vi "Process.vi"(8 "error in":errorcluster, 11 "System":refnum<class "System.lvclass">) -> (0 "error out":errorcluster, 3 "System out":refnum<class "System.lvclass">)   [LabVIEW 2014, in "System.lvclass"]
doc: "JKI State Machine Objects (SMO) 1.4.0.57\nJKI - JKI\nCopyright (c) 2018, JKI"
uses:
  System.lvclass
  <vilib>/JKI/JKI SMO/SMO/Typedefs/Parent Call--Enum.ctl
  Pump class/Pump State - cluster.ctl
  System.lvclass/System.ctl
  Pump class/Pump.lvclass/Pump.ctl
  <vilib>/JKI/JKI SMO/SMO/SMO.lvclass
  Pump class/Pump.lvclass
panel:
  in  "Speed Command":dbl
  in  "Change Pump Speed":bool
  out "Pump State":T1(graph)
  # "For instructions on how to use the JKI State Machine Objects, examples and video tutorials, visit:\nhttp://jki.net/state-machine-objects/\n\nJKI State Machine Objects™\nhttp://jki.net/state-machine-objects/\nCopyright (C) 2005-2015, JKI <info@jki.net>\nALL RIGHTS RESERVED"
  # "SYSTEM PROCESS USER INTERFACE"
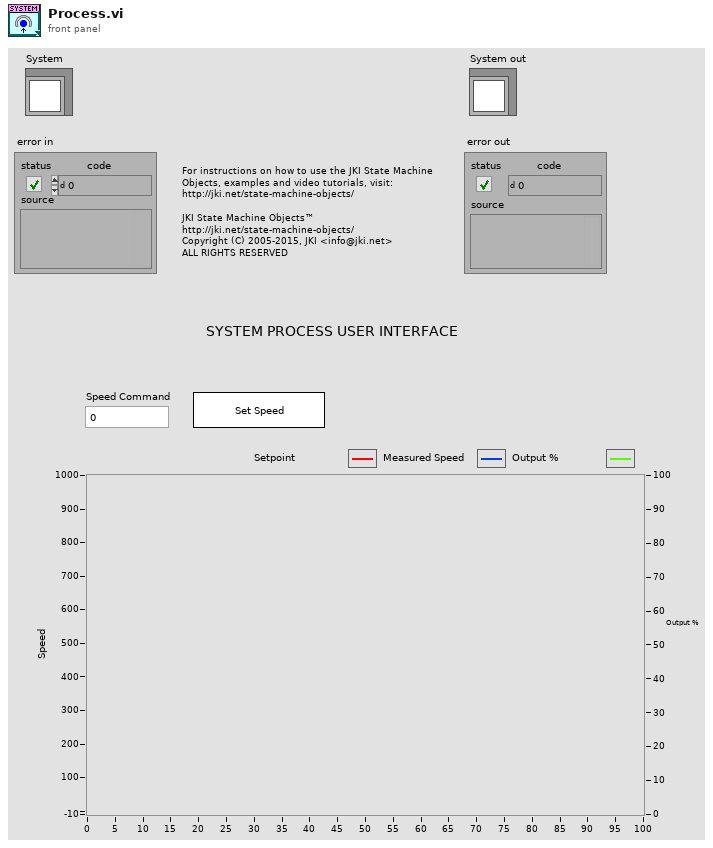
[diagram p1: front panel]
types:
  T1 = typedef "Pump.lvclass/Pump State - cluster.ctl" = cluster{"Pump Setpoint":dbl, "Pump Speed":dbl, "Output %":dbl}
  T2 = typedef "SMO.lvclass/Parent Call--Enum.ctl" = enum16{"Allows parent to run", "Does not request parent to run"}
  T3 = enum32{"invalid app kind", "Development System", "Run Time System", "Student Edition", "Embedded LabVIEW", "Evaluation", "Custom"}
  T4 = enum32{"Invalid", "Standard", "Closed", "Hidden", "Minimized", "Maximized"}
  T5 = cluster{"Core":cluster{"Current VI Reference":refnum<vi>, "Close Panel on Exit?":bool, "error":errorcluster}, "Self Reference":refnum<class "System.lvclass">}
  T6 = cluster{"Current VI Reference":refnum<vi>, "Close Panel on Exit?":bool, "error":errorcluster}
  T7 = typedef "SMO.lvclass/Protected Events.ctl" = cluster{"StopProcesses":refnum<user-event>, "AbortProcesses":refnum<user-event>, "Config Changed":refnum<user-event>, "Dependency":refnum<user-event>}
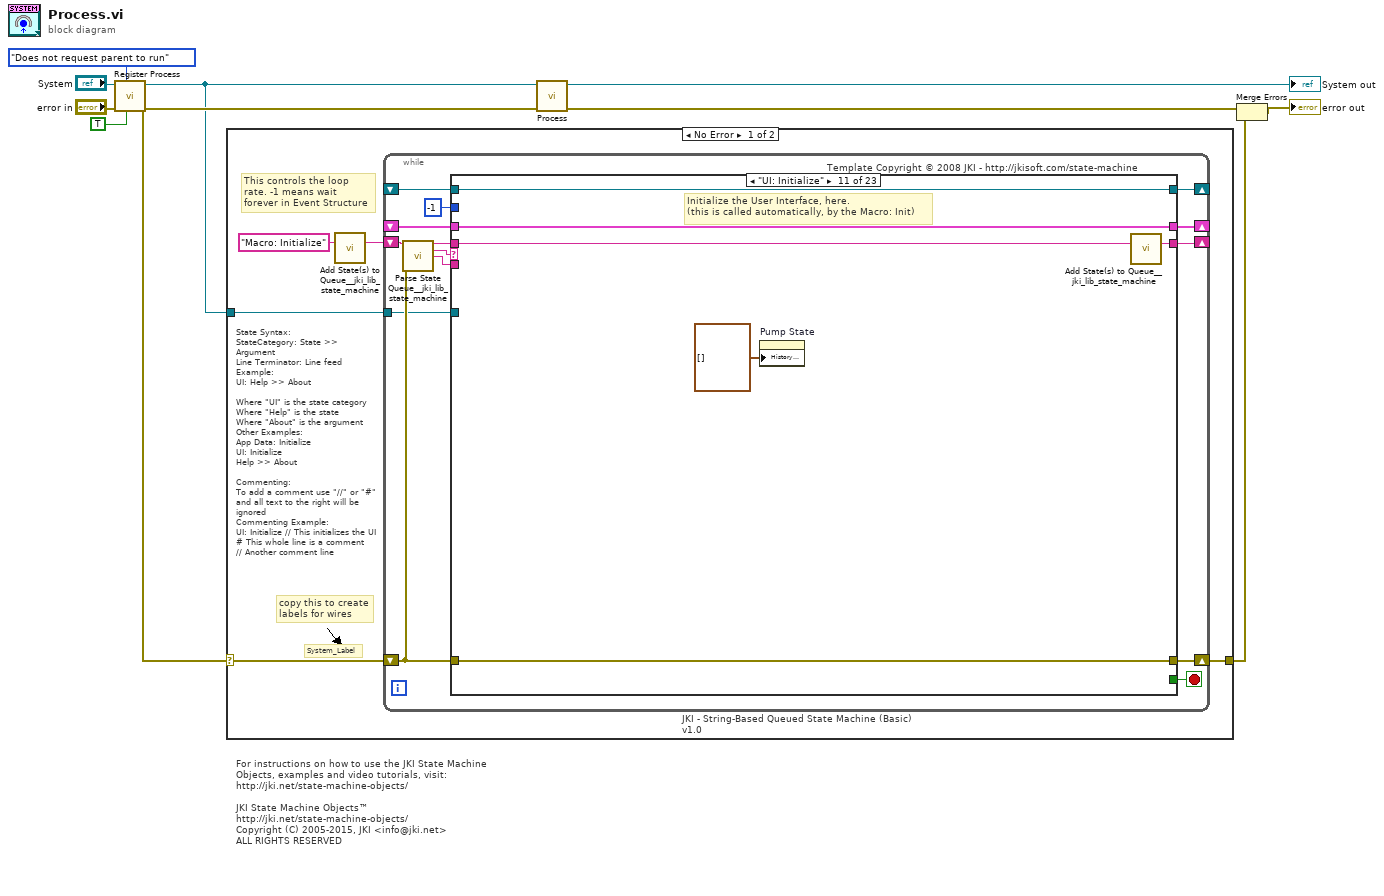
[diagram p0: block diagram]
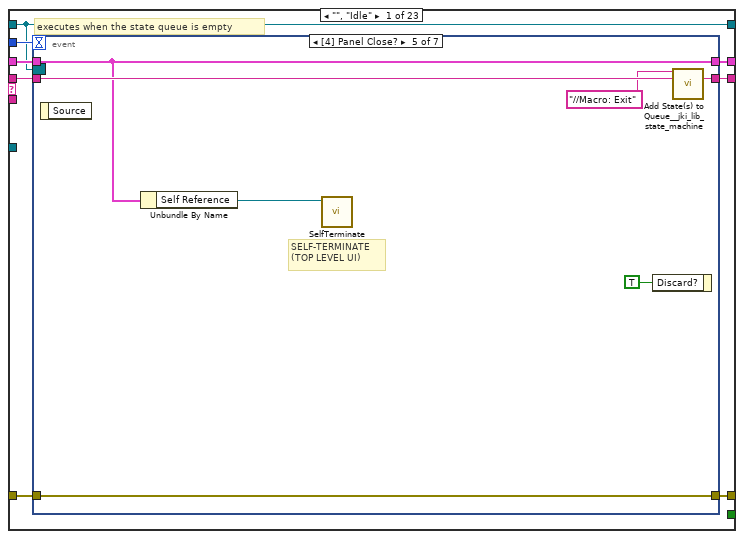
[diagram p2: hidden frame]
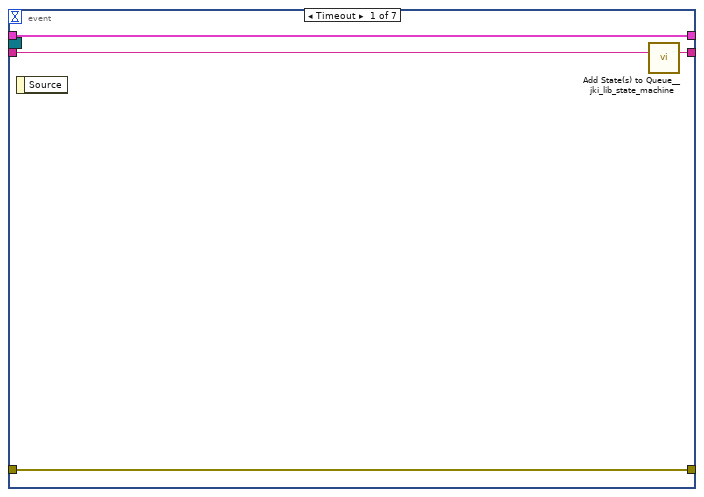
[diagram p3: hidden frame]
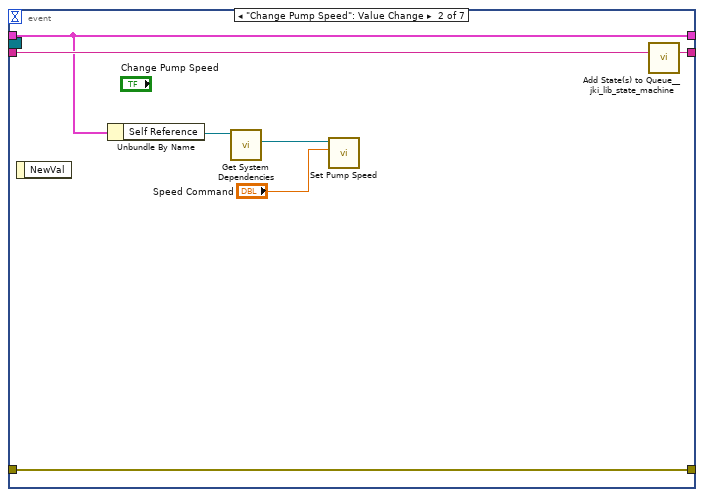
[diagram p4: hidden frame]
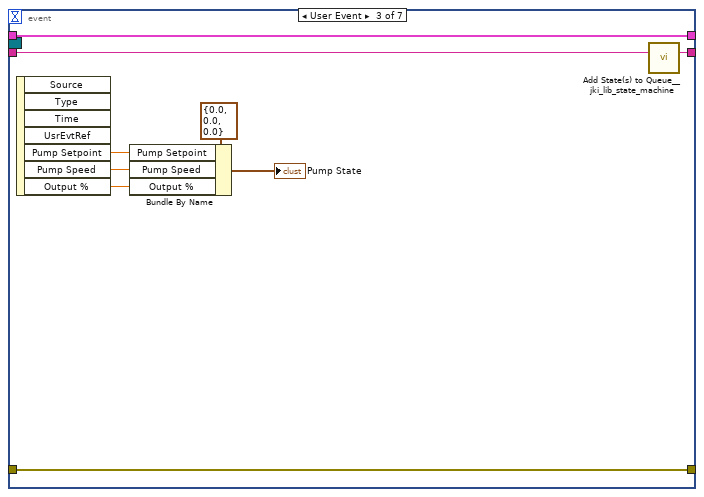
[diagram p5: hidden frame]
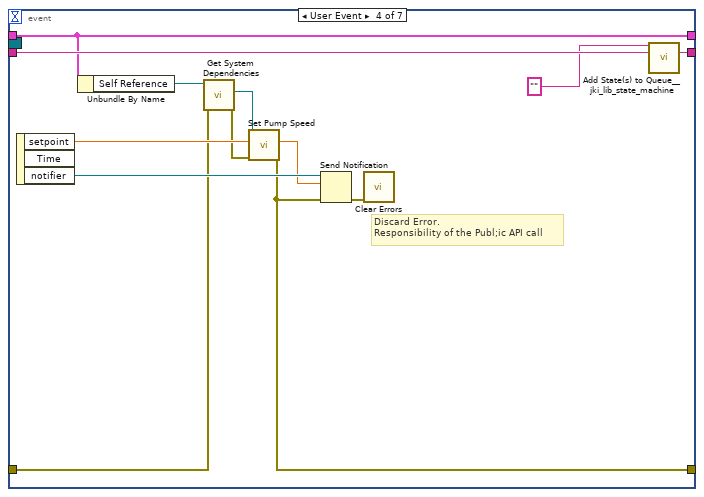
[diagram p6: hidden frame]
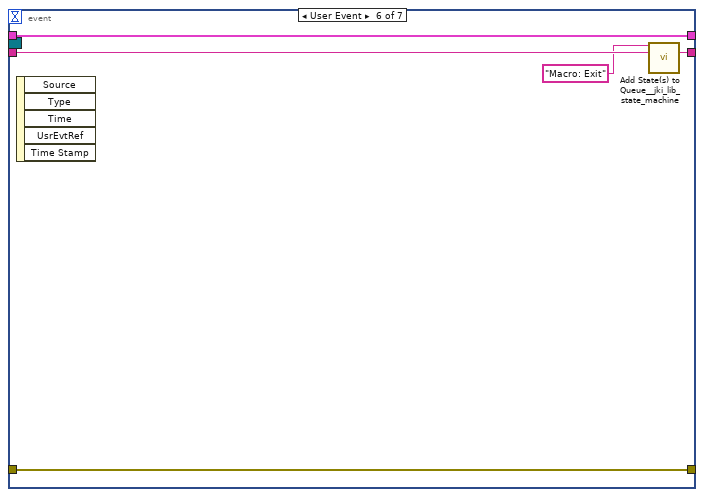
[diagram p7: hidden frame]
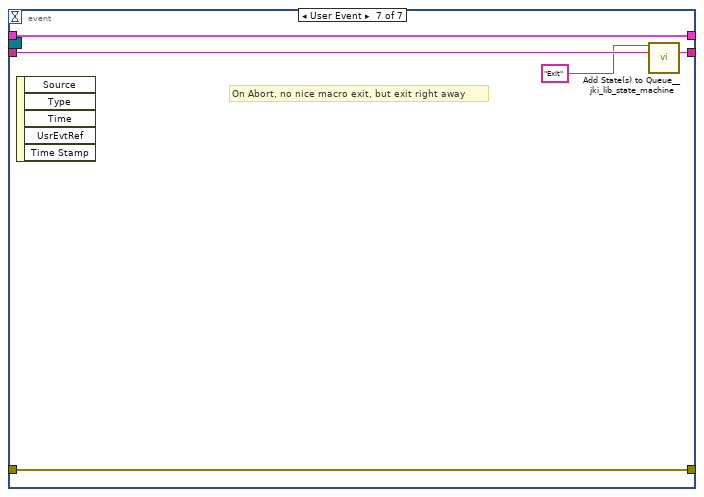
[diagram p8: hidden frame]
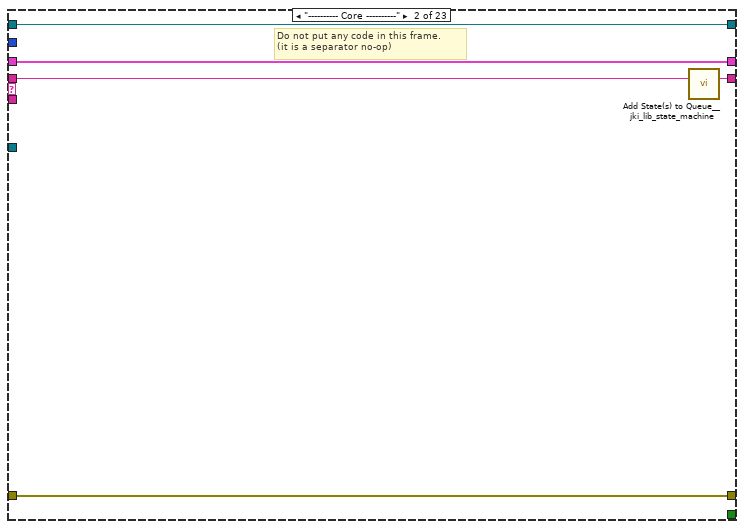
[diagram p9: hidden frame]
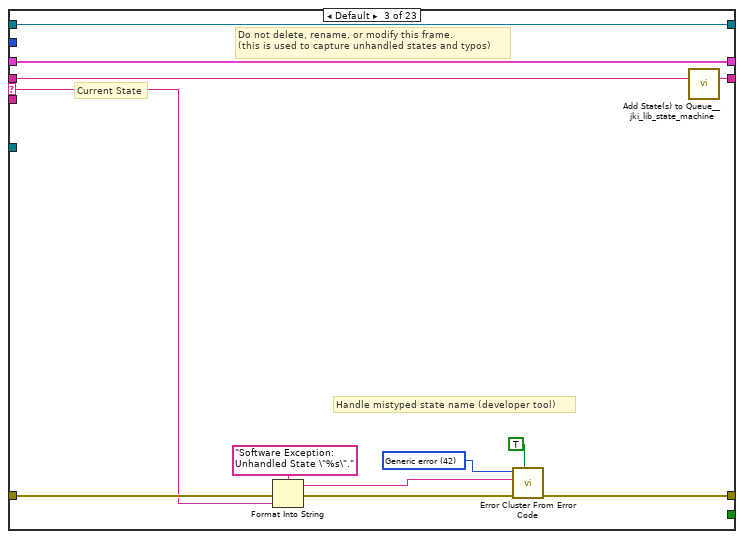
[diagram p10: hidden frame]
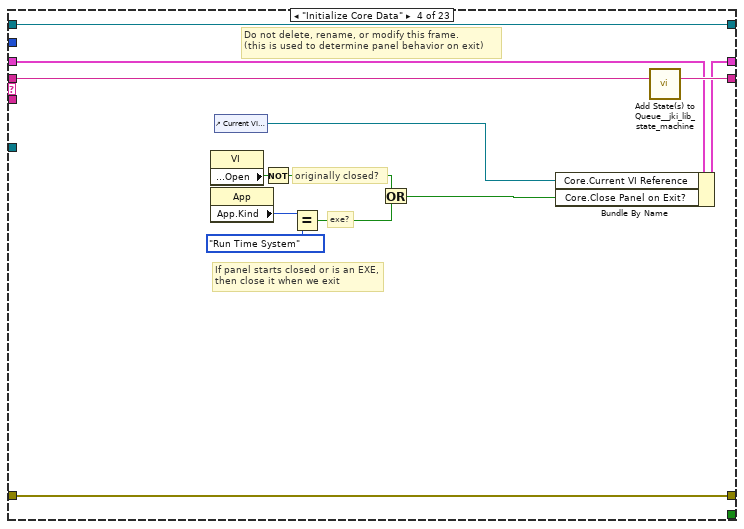
[diagram p11: hidden frame]
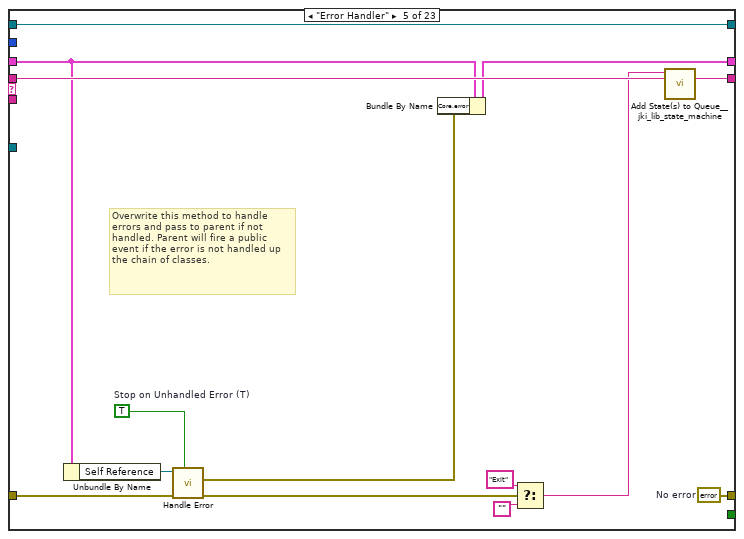
[diagram p12: hidden frame]
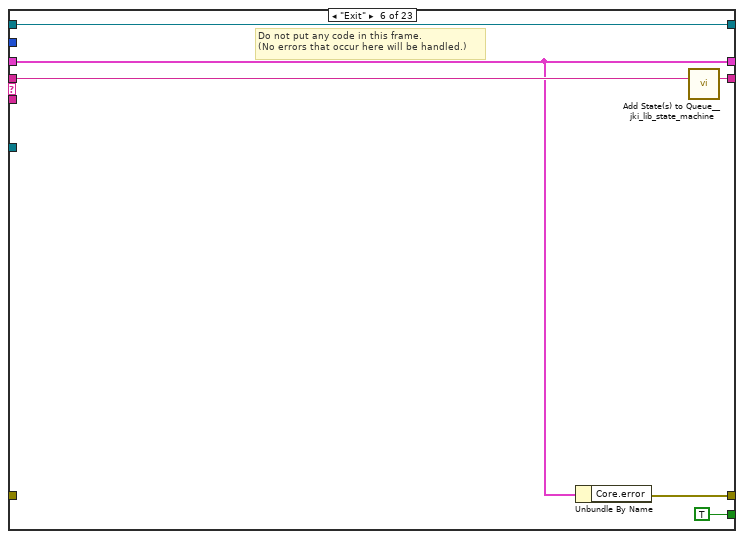
[diagram p13: hidden frame]
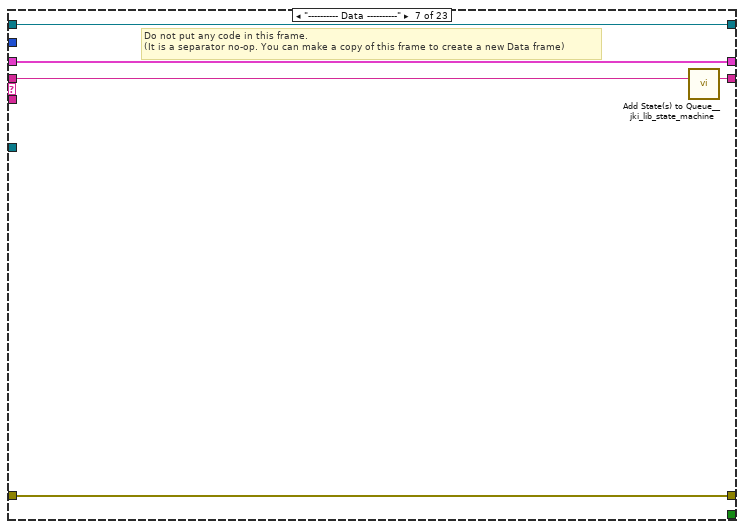
[diagram p14: hidden frame]
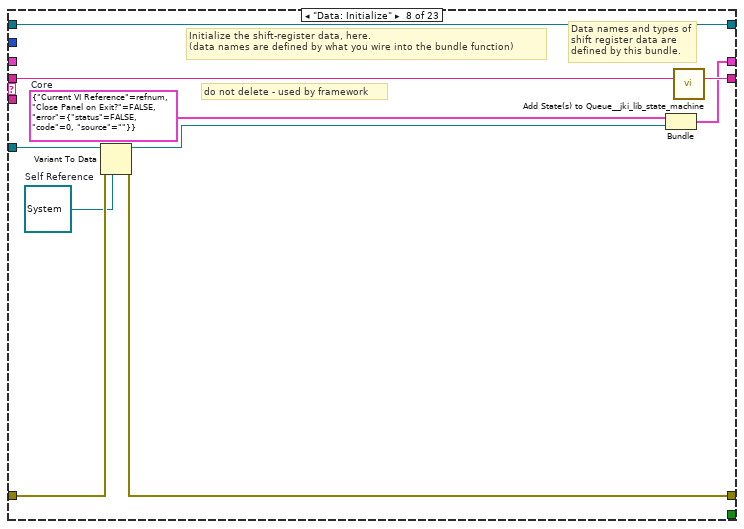
[diagram p15: hidden frame]
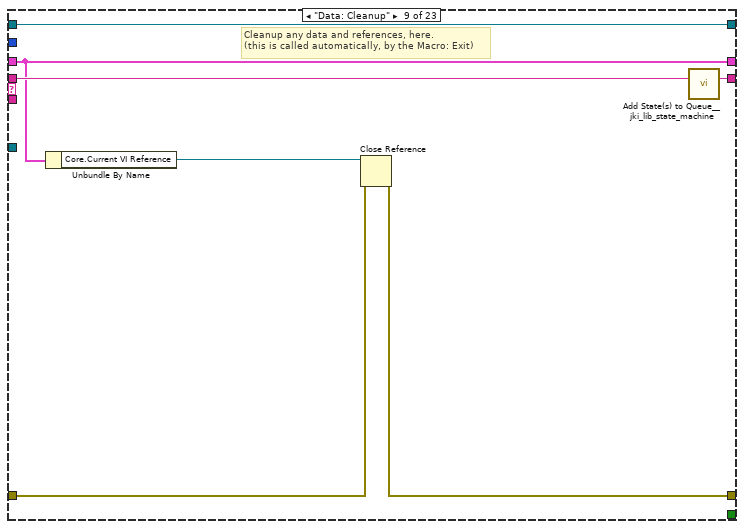
[diagram p16: hidden frame]
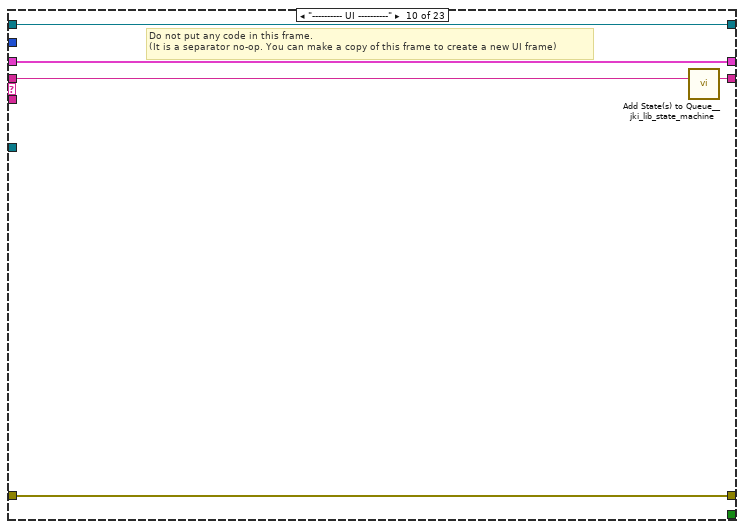
[diagram p17: hidden frame]
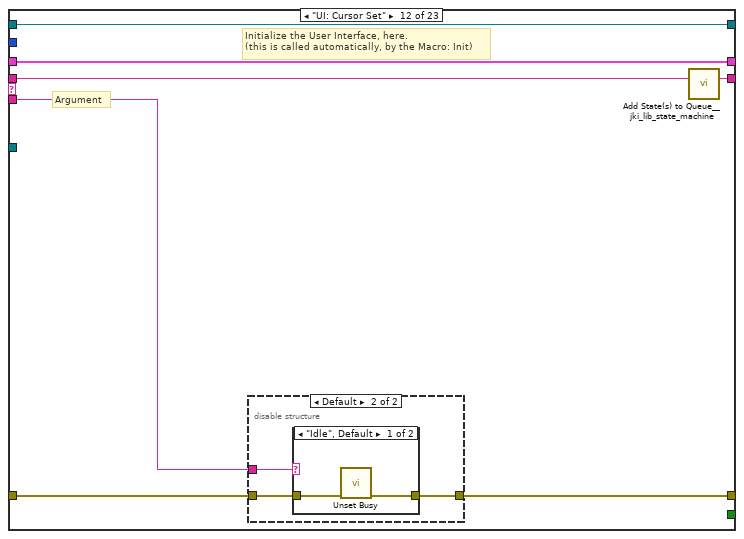
[diagram p18: hidden frame]
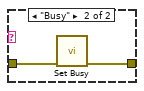
[diagram p20: hidden frame]
diagram:
  # "For instructions on how to use the JKI State Machine Objects, examples and video tutorials, visit:\nhttp://jki.net/state-machine-objects/\n\nJKI State Machine Objects™\nhttp://jki.net/state-machine-objects/\nCopyright (C) 2005-2015, JKI <info@jki.net>\nALL RIGHTS RESERVED"
  n1 = call <vilib>:"Register Process.vi"("Forces Self to Run (F)"=TRUE, "Parent Call"=Parent_Call--Enum."Does not request parent to run", "error in (no error)"="error in", "SMO"="System") -> ("error out"=w10:errorcluster, "SMO out"=w9:refnum<class "System.lvclass">)  [unwired: 6 in]
  n2 = case shown="No Error" w10 {
    selector: w10 -> [w12 w302]
    tunnel: w9 -> [w13 _]
    tunnel: [w11 w302] -> w7
    frame No Error {
      # "State Syntax:\nStateCategory: State >> Argument\nLine Terminator: Line feed\nExample:\nUI: Help >> About\n\nWhere \"UI\" is the state category\nWhere \"Help\" is the state\nWhere \"About\" is the argument\nOther Examples:\nApp Data: Initialize\nUI: Initialize\nHelp >> About\n\nCommenting:\nTo add a comment use \"//\" or \"#\" and all text to the right will be ignored\nCommenting Example:\nUI: Initialize // This initializes the UI\n# This whole line is a comment\n// Another comment line"
      # "copy this to create labels for wires"
      # "This controls the loop rate. -1 means wait forever in Event Structure"
      # "System_Label"
      n3 = call <vilib>:"Add State(s) to Queue__jki_lib_state_machine.vi"("State(s) in (\"\")"="Macro: Initialize") -> ("States Out"=w15:string)  [unwired: 14 in]
      n4 = while "JKI - String-Based Queued State Machine (Basic) v1.0" {
        shift-right: [w22] -> _
        shift-left: _ -> [w21]
        shift-right: [w25] -> w11
        shift-left: w12 -> [w19]
        shift-right: [w24] -> _
        shift-left: w15 -> [w26]
        tunnel: w13 -> [w18]
        shift-right: [w17] -> _
        shift-left: _ -> [w16]
        stop <- w23 stop-if-true
        # "Template Copyright © 2008 JKI - http://jkisoft.com/state-machine"
        n5 = call <vilib>:"Parse State Queue__jki_lib_state_machine.vi"("State Queue"=w26, "Error In (no error)"=w19) -> ("Remaining States"=w28:string, "Current State"=w29:string, "Arguments"=w27:string)  [unwired: 11 in]
        n6 = case shown="\"UI: Initialize\"" w29 {
          selector: w29 -> [_ _ w94 _ _ _ _ _ _ _ _ _ _ _ _ _ _ _ _ _ _ _ _]
          tunnel: w28 -> [w37 w92 w98 w117 w131 w137 w142 w152 w159 w164 w170 w177 w193 w225 w234 w240 w254 w259 w270 w275 w290 w296 w301]
          tunnel: w27 -> [_ _ _ _ _ _ _ _ _ _ _ w171 w187 _ _ _ _ _ _ _ _ _ _]
          tunnel: w21 -> [w35 w89 w96 w108 w125 w133 w139 _ w154 w161 w168 w175 w189 w222 w230 w236 w245 w256 w267 w272 w288 w294 w299]
          tunnel: [w34 w90 w100 w114 w126 w132 w140 w148 w155 w162 w167 w172 w190 w223 w232 w238 w252 w257 w261 w273 w285 w292 w297] -> w25
          tunnel: w19 -> [w33 w90 w99 w114 w127 _ w140 w149 w156 w162 w167 w173 w191 w223 w232 w238 w252 w257 w262 w273 w286 w292 w297]
          tunnel: [w36 w91 w97 w116 w130 w136 w141 w151 w158 w163 w169 w176 w192 w224 w233 w239 w253 w258 w269 w274 w289 w295 w300] -> w24
          tunnel: [_ _ _ _ _ TRUE _ _ _ _ _ _ _ _ _ _ _ _ _ _ _ _ _] -> w23
          tunnel: [w32 w89 w96 w115 w124 w133 w139 w150 w154 w161 w168 w175 w189 w222 w230 w236 w245 w256 w267 w272 w288 w294 w299] -> w22
          tunnel: -1 ("Timeout") -> [w31 _ _ _ _ _ _ _ _ _ _ _ _ _ _ _ _ _ _ _ _ _ _]
          tunnel: w18 -> [_ _ _ _ _ _ _ w147 _ _ _ _ _ _ _ _ _ _ _ _ _ _ _]
          tunnel: [w30 w88 w93 w105 w129 w134 w138 w145 w153 w160 w166 w174 w186 w221 w231 w237 w246 w255 w268 w271 w281 w293 w298] -> w17
          tunnel: w16 -> [w30 w88 w93 w105 w129 w134 w138 w145 w153 w160 w166 w174 w186 w221 w231 w237 w246 w255 w268 w271 _ w293 w298]
          frame "", "Idle" {
            # "executes when the state queue is empty"
            n7 = event shown="[4] Panel Close?" {
              selector: w30 -> [_ _ _ _ _ _ _]
              dyn-events: _ -> [_ _ _ _ _ _ _]
              timeout: w31 -> [_ _ _ _ _ _ _]
              tunnel: w37 -> [w41 w48 w57 w70 w77 w82 w87]
              tunnel: [w40 w47 w56 w69 w76 w81 w86] -> w36
              tunnel: w35 -> [w39 w45 w55 w68 w72 w79 w84]
              tunnel: [w38 w46 w54 w58 w75 w80 w85] -> w34
              tunnel: w33 -> [w38 w46 w54 w59 w75 w80 w85]
              tunnel: [w39 w45 w55 w68 w72 w79 w84] -> w32
              event Timeout {
                n8 = event-data() -> ()  [unwired: 1 in, 1 out]
                n9 = call <vilib>:"Add State(s) to Queue__jki_lib_state_machine.vi"("State(s) in (\"\")"=w41) -> ("States Out"=w40:string)  [unwired: 14 in]
              }
              event "Change Pump Speed": Value Change {
                n10 = event-data() -> ()  [unwired: 1 in, 1 out]
                n11 = Unbundle By Name(w45) -> ("Self Reference"=w44:refnum<class "System.lvclass">)
                n12 = call "Get System Dependencies.vi"("System in"=w44) -> ("Pump"=w43:refnum<class "Pump.lvclass">)  [unwired: 8 in, 2 out]
                n13 = call "Set Pump Speed.vi"("Speed Command"="Speed Command", "Pump in"=w43) -> ()  [unwired: 6 in, 4 out]
                n14 = call <vilib>:"Add State(s) to Queue__jki_lib_state_machine.vi"("State(s) in (\"\")"=w48) -> ("States Out"=w47:string)  [unwired: 14 in]
              }
              event User Event {
                n15 = event-data() -> ("Pump Setpoint"=w52:dbl, "Pump Speed"=w51:dbl, "Output %"=w50:dbl)  [unwired: 1 in, 4 out]
                n16 = Bundle By Name(cluster=T1 {"Pump Setpoint"=0.0, "Pump Speed"=0.0, "Output %"=0.0} ("Pump State"), "Pump Setpoint"=w52, "Pump Speed"=w51, "Output %"=w50) -> (→"Pump State":T1)
                n17 = call <vilib>:"Add State(s) to Queue__jki_lib_state_machine.vi"("State(s) in (\"\")"=w57) -> ("States Out"=w56:string)  [unwired: 14 in]
              }
              event User Event {
                # "Discard Error.\nResponsibility of the Publ;ic API call"
                n18 = event-data() -> ("setpoint"=w64:dbl, "notifier"=w63:refnum<notifier>)  [unwired: 1 in, 1 out]
                n19 = Unbundle By Name(w68) -> ("Self Reference"=w66:refnum<class "System.lvclass">)
                n20 = call "Get System Dependencies.vi"("error in (no error)"=w59, "System in"=w66) -> ("error out"=w61:errorcluster, "Pump"=w65:refnum<class "Pump.lvclass">)  [unwired: 7 in, 1 out]
                n21 = call "Set Pump Speed.vi"("error in (no error)"=w61, "Speed Command"=w64, "Pump in"=w65) -> ("error out"=w58:errorcluster, "Pump Setpoint"=w62:dbl)  [unwired: 5 in, 2 out]
                n22 = Send Notification(notification=w62, notifier=w63, error in (no error)=w58) -> (error out=w60:errorcluster)  [unwired: 1 out]
                n23 = call <vilib>:"Clear Errors.vi"("error in (no error)"=w60) -> ()  [unwired: 5 in, 2 out]
                n24 = call <vilib>:"Add State(s) to Queue__jki_lib_state_machine.vi"("State(s) in Front (\"\")"="" ("t"), "State(s) in (\"\")"=w70) -> ("States Out"=w69:string)  [unwired: 13 in]
              }
              event Panel Close? {
                # "SELF-TERMINATE\n(TOP LEVEL UI)"
                n25 = event-data() -> ()  [unwired: 1 in, 1 out]
                n26 = Unbundle By Name(w72) -> ("Self Reference"=w71:refnum<class "System.lvclass">)
                n27 = call <vilib>:"SelfTerminate.vi"("SMO in"=w71) -> ()  [unwired: 9 in, 2 out]
                n28 = event-data("Discard?"=TRUE) -> ()  [unwired: 1 in, 1 out]
                n29 = call <vilib>:"Add State(s) to Queue__jki_lib_state_machine.vi"("State(s) in Front (\"\")"="//Macro: Exit", "State(s) in (\"\")"=w77) -> ("States Out"=w76:string)  [unwired: 13 in]
              }
              event User Event {
                n30 = event-data() -> ()  [unwired: 1 in, 5 out]
                n31 = call <vilib>:"Add State(s) to Queue__jki_lib_state_machine.vi"("State(s) in Front (\"\")"="Macro: Exit", "State(s) in (\"\")"=w82) -> ("States Out"=w81:string)  [unwired: 13 in]
              }
              event User Event {
                # "On Abort, no nice macro exit, but exit right away"
                n32 = event-data() -> ()  [unwired: 1 in, 5 out]
                n33 = call <vilib>:"Add State(s) to Queue__jki_lib_state_machine.vi"("State(s) in Front (\"\")"="Exit", "State(s) in (\"\")"=w87) -> ("States Out"=w86:string)  [unwired: 13 in]
              }
            }
          }
          frame "---------- Core ----------" {
            # "Do not put any code in this frame.\n(it is a separator no-op)"
            n34 = call <vilib>:"Add State(s) to Queue__jki_lib_state_machine.vi"("State(s) in (\"\")"=w92) -> ("States Out"=w91:string)  [unwired: 14 in]
          }
          frame Default {
            w103 = 42 items=["No error", "Argument error", "Memory is full", "Out of zone", "End of file", "File already open", "Generic file I/O error", "File not found", "File permission error", "Disk is full", "Duplicate path", "Too many files open", "System feature not enabled", "Resource file not found", "Cannot add resource", "Resource not found", "Image not found", "Image memory error", "Pen does not exist", "Config type invalid", "Config token not found", "Config parse error", "Config memory error", "Bad external code format", "Bad external code offset", "External code not present", "Null window", "Destroy window error", "Null menu", "Print aborted", "Bad print record", "Print driver error", "Windows error during printing", "Memory error during printing", "Print dialog error", "Generic print error", "Invalid device refnum", "Device not found", "Device parameter error", "Device unit error", "Cannot open device", "Device call aborted", "Generic error", "Cancelled by user", "Object ID too low", "Object ID too high", "Object not in heap", "Unknown heap", "Unknown object (invalid DefProc)", "Unknown object (DefProc not in table)", "Message out of range", "Invalid (null) method", "Unknown message", "Manager call not supported", "Bad address", "Network operation in progress", "Network operation timed out", "Connection is busy", "Network attribute not supported", "Network error", "Address in use", "System out of memory", "Connection aborted", "Connection refused", "Not connected", "Already connected", "Connection closed", "Initialization error (interapplication manager)", "Bad occurrence", "Wait on unbound occurrence handler", "Occurrence queue overflow", "Datalog type conflict", "Unused", "Unrecognized type (interapplication manager)", "Memory corrupt", "Failed to make temporary DLL", "Old CIN version", "Drag socket not found", "Failed to load drop-object", "Failed to register OLE object", "Failed to release OLE object", "Format specifier type mismatch", "Unknown format specifier", "Too few format specifiers", "Too many format specifiers", "Scan failed", "Newer CIN version", "Error converting to variant", "Runtime menu error", "Password tampered", "Variant attribute not found", "Incompatible variant data type", "Event data is not available", "Event Store is not present", "Occurrence is not found", "Event Queue is not created", "Event info is not available", "Refnum passed is NULL", "Error retrieving Class GUID", "Error retrieving CoClass GUID", "Error retrieving TypeLib GUID.", "Bad built application magic bytes.", "Specific driver is different from the specific driver associated with the Logical Name.", "There is no session opened to the class driver.", "Max Error", "MAX - Error with config objects", "MAX - Error loading configuration", "MAX - Group not supported"]
            # "Current State"
            # "Do not delete, rename, or modify this frame.\n(this is used to capture unhandled states and typos)"
            # "Handle mistyped state name (developer tool)"
            n35 = Format Into String(format string="Software Exception: Unhandled State \"%s\"." ("message"), error in=w99, w94) -> (resulting string=w102:string, error out=w101:errorcluster)  [unwired: 1 in]
            n36 = call <vilib>:"Error Cluster From Error Code.vi"("show call chain? (False)"=TRUE, "error in (no error)"=w101, "error message (\"\")"=w102, "error code (0)"=w103) -> ("error out"=w100:errorcluster)  [unwired: 5 in]
            n37 = call <vilib>:"Add State(s) to Queue__jki_lib_state_machine.vi"("State(s) in (\"\")"=w98) -> ("States Out"=w97:string)  [unwired: 14 in]
          }
          frame "Initialize Core Data" {
            # "Do not delete, rename, or modify this frame.\n(this is used to determine panel behavior on exit)"
            # "originally closed?"
            # "exe?"
            # "If panel starts closed or is an EXE, then close it when we exit"
            n38 = property class="VI"() -> ("Front Panel.Open"=w113:bool)  [unwired: 2 in, 2 out]
            n39 = property class="App"() -> ("App.Kind"=w112:T3)  [unwired: 2 in, 2 out]
            n40 = control-ref of="Current VI Reference"() -> (w106:refnum<vi>)
            n41 = Not(x=w113) -> (.not. x?=w110:bool)
            n42 = Equal?(x=w112, y=T3."Run Time System" ("Application:Kind")) -> (x = y?=w109:bool)
            n43 = Or(x=w110, y=w109) -> (x .or. y?=w107:bool)
            n44 = Bundle By Name(cluster=w108, "Core.Current VI Reference"=w106, "Core.Close Panel on Exit?"=w107) -> (w115:T5)
            n45 = call <vilib>:"Add State(s) to Queue__jki_lib_state_machine.vi"("State(s) in (\"\")"=w117) -> ("States Out"=w116:string)  [unwired: 14 in]
          }
          frame "Error Handler" {
            w118 = TRUE  # Stop on Unhandled Error (T)
            w126 = errorcluster {"status"=FALSE, "code"=0, "source"=""}  # No error
            # "Overwrite this method to handle errors and pass to parent if not handled. Parent will fire a public event if the error is not handled up the chain of classes."
            n46 = Unbundle By Name(w125) -> ("Self Reference"=w128:refnum<class "System.lvclass">)
            n47 = call-dynamic "Handle Error.vi"("Stop on Unhandled Error (T)"=w118, "error in"=w127, "SMO"=w128) -> ("handling error"=w119:errorcluster, "Unhandled error"=w122:errorcluster)  [unwired: 6 in, 1 out]
            n48 = Bundle By Name(cluster=w125, "Core.error"=w122) -> (w124:T5)
            n49 = Select(t="Exit", s=w119, f="") -> (s? t:f=w123:string)
            n50 = call <vilib>:"Add State(s) to Queue__jki_lib_state_machine.vi"("State(s) in Front (\"\")"=w123, "State(s) in (\"\")"=w131) -> ("States Out"=w130:string)  [unwired: 13 in]
          }
          frame "Exit" {
            # "Do not put any code in this frame.\n(No errors that occur here will be handled.)"
            n51 = Unbundle By Name(w133) -> ("Core.error"=w132:errorcluster)
            n52 = call <vilib>:"Add State(s) to Queue__jki_lib_state_machine.vi"("State(s) in (\"\")"=w137) -> ("States Out"=w136:string)  [unwired: 14 in]
          }
          frame "---------- Data ----------" {
            # "Do not put any code in this frame.\n(It is a separator no-op. You can make a copy of this frame to create a new Data frame)"
            n53 = call <vilib>:"Add State(s) to Queue__jki_lib_state_machine.vi"("State(s) in (\"\")"=w142) -> ("States Out"=w141:string)  [unwired: 14 in]
          }
          frame "Data: Initialize" {
            w143 = refnum<class "System.lvclass"> refnum  # Self Reference
            w144 = T6 {"Current VI Reference"=refnum, "Close Panel on Exit?"=FALSE, "error"={"status"=FALSE, "code"=0, "source"=""}}  # Core
            # "do not delete - used by framework"
            # "Data names and types of shift register data are defined by this bundle."
            # "Initialize the shift-register data, here.\n(data names are defined by what you wire into the bundle function)"
            n54 = Variant To Data(error in=w149, type=w143, Variant=w147) -> (data=w146:refnum<class "System.lvclass">, error out=w148:errorcluster)
            n55 = Bundle("Core"=w144, "Self Reference"=w146) -> (w150:T5)  [unwired: 1 in]
            n56 = call <vilib>:"Add State(s) to Queue__jki_lib_state_machine.vi"("State(s) in (\"\")"=w152) -> ("States Out"=w151:string)  [unwired: 14 in]
          }
          frame "Data: Cleanup" {
            # "Cleanup any data and references, here.\n(this is called automatically, by the Macro: Exit)"
            n57 = Unbundle By Name(w154) -> ("Core.Current VI Reference"=w157:refnum<vi>)
            n58 = Close Reference(reference=w157, error in (no error)=w156) -> (error out=w155:errorcluster)
            n59 = call <vilib>:"Add State(s) to Queue__jki_lib_state_machine.vi"("State(s) in (\"\")"=w159) -> ("States Out"=w158:string)  [unwired: 14 in]
          }
          frame "---------- UI ----------" {
            # "Do not put any code in this frame.\n(It is a separator no-op. You can make a copy of this frame to create a new UI frame)"
            n60 = call <vilib>:"Add State(s) to Queue__jki_lib_state_machine.vi"("State(s) in (\"\")"=w164) -> ("States Out"=w163:string)  [unwired: 14 in]
          }
          frame "UI: Initialize" {
            # "Initialize the User Interface, here.\n(this is called automatically, by the Macro: Init)"
            n61 = property on="Pump State" class="WFChart (strict)"("History Data"=T1[] []) -> ()  [unwired: 2 in, 2 out]
            n62 = call <vilib>:"Add State(s) to Queue__jki_lib_state_machine.vi"("State(s) in (\"\")"=w170) -> ("States Out"=w169:string)  [unwired: 14 in]
          }
          frame "UI: Cursor Set" {
            # "Argument"
            # "Initialize the User Interface, here.\n(this is called automatically, by the Macro: Init)"
            n63 = disable-structure shown="Default" {
              disable-tunnel: w173 -> [w178 w181]
              disable-tunnel: [w178 w180] -> w172
              disable-tunnel: w171 -> [_ w179]
              frame condition #0 {
              }
              frame condition #1 (active) {
                n64 = case shown="\"Idle\", Default" w179 {
                  tunnel: w181 -> [w183 w185]
                  tunnel: [w182 w184] -> w180
                  frame "Idle", Default {
                    n65 = call <vilib>:"Unset Busy.vi"("error in (no error)"=w183) -> ("error out"=w182:errorcluster)  [unwired: 10 in]
                  }
                  frame "Busy" {
                    n66 = call <vilib>:"Set Busy.vi"("error in (no error)"=w185) -> ("error out"=w184:errorcluster)  [unwired: 9 in, 1 out]
                  }
                }
              }
            }
            n67 = call <vilib>:"Add State(s) to Queue__jki_lib_state_machine.vi"("State(s) in (\"\")"=w177) -> ("States Out"=w176:string)  [unwired: 14 in]
          }
          frame "UI: Front Panel State" {
            # "Argument"
            # "Set Front Panel Open or Closed\n(Usage: \"UI: Front Panel State >> Open|Close\")"
            n68 = Unbundle By Name(w189) -> ("Core.Current VI Reference"=w188:refnum<vi>)
            n69 = disable-structure shown="Default" {
              disable-tunnel: w191 -> [w197 w220]
              disable-tunnel: [w196 w220] -> w190
              disable-tunnel: w188 -> [w195 _]
              disable-tunnel: w187 -> [w194 _]
              frame condition #0 (active) {
                n70 = case shown="\"Close\"" w194 {
                  tunnel: w197 -> [w201 w214]
                  tunnel: [w203 w215] -> w196
                  tunnel: w195 -> [w202 w212]
                  frame "Open", Default {
                    n71 = property class="VI"(reference=w202, error in=w201) -> (reference out=w199:refnum<vi>, error out=w200:errorcluster, "FP.State"=w198:T4)
                    n72 = case shown="\"Closed\"" w198 {
                      tunnel: [w206 w209] -> w203
                      tunnel: w200 -> [w205 w209]
                      tunnel: w199 -> [w204 _]
                      frame "Closed" {
                        n73 = invoke class="VI" method="FP.Open"(reference=w204, error in=w205, "Activate"=TRUE, "State"=T4."Standard") -> (error out=w206:errorcluster)  [unwired: 1 in, 4 out]
                      }
                      frame Default {
                      }
                    }
                  }
                  frame "Close" {
                    n74 = property class="VI"(reference=w212, error in=w214) -> (reference out=w211:refnum<vi>, error out=w213:errorcluster, "FP.State"=w210:T4)
                    n75 = case shown="Default" w210 {
                      tunnel: [w216 w219] -> w215
                      tunnel: w213 -> [w216 w218]
                      tunnel: w211 -> [_ w217]
                      frame "Invalid", "Closed" {
                      }
                      frame Default {
                        n76 = invoke class="VI" method="FP.Close"(reference=w217, error in=w218) -> (error out=w219:errorcluster)  [unwired: 1 in, 2 out]
                      }
                    }
                  }
                }
              }
              frame condition #1 {
              }
            }
            n77 = call <vilib>:"Add State(s) to Queue__jki_lib_state_machine.vi"("State(s) in (\"\")"=w193) -> ("States Out"=w192:string)  [unwired: 14 in]
          }
          frame "---------- Macro ----------" {
            # "Do not put any code in this frame.\n(It is a separator no-op. You can make a copy of this frame to create a new Macro frame)"
            n78 = call <vilib>:"Add State(s) to Queue__jki_lib_state_machine.vi"("State(s) in (\"\")"=w225) -> ("States Out"=w224:string)  [unwired: 14 in]
          }
          frame "Macro: Initialize" {
            w228 = "UI: Initialize\nUI: Front Panel State >> Open"  # UI: Initialize UI: Front Panel State >> Open
            # "Initialization Macro\n(This is called once, when the VI starts)"
            n79 = call <vilib>:"Add State(s) to Queue__jki_lib_state_machine.vi"("State(s) in Front (\"\")"="Data: Initialize\nInitialize Core Data\nEvents: Register", "State(s) in (\"\")"="Process: Sync", "State(s) at Back (\"\")"=w228) -> ("States Out"=w227:string)  [unwired: 12 in]
            n80 = call <vilib>:"Add State(s) to Queue__jki_lib_state_machine.vi"("State(s) in Front (\"\")"=w227, "State(s) in (\"\")"=w234) -> ("States Out"=w233:string)  [unwired: 13 in]
          }
          frame "Macro: Process Queue" {
            n81 = call <vilib>:"Add State(s) to Queue__jki_lib_state_machine.vi"("State(s) in Front (\"\")"="", "State(s) in (\"\")"=w240) -> ("States Out"=w239:string)  [unwired: 13 in]
          }
          frame "Macro: Exit" {
            # "Exit Macro\n(This is called once, when the VI exits)"
            n82 = Unbundle By Name(w245) -> ("Core.Close Panel on Exit?"=w251:bool)
            n83 = Select(t="UI: Front Panel State >> Close", s=w251, f="") -> (s? t:f=w248:string)
            n84 = call <vilib>:"Add State(s) to Queue__jki_lib_state_machine.vi"("State(s) in Front (\"\")"="Data: Cleanup\nEvents: Unregister", "State(s) in (\"\")"="Process: Sync", "State(s) at Back (\"\")"="Exit") -> ("States Out"=w242:string)  [unwired: 12 in]
            n85 = call <vilib>:"Add State(s) to Queue__jki_lib_state_machine.vi"("State(s) in (\"\")"=w248, "State(s) at Back (\"\")"=w242) -> ("States Out"=w247:string)  [unwired: 13 in]
            n86 = call <vilib>:"Add State(s) to Queue__jki_lib_state_machine.vi"("State(s) in Front (\"\")"=w247, "State(s) in (\"\")"=w254) -> ("States Out"=w253:string)  [unwired: 13 in]
          }
          frame "---------- Process ----------" {
            # "Template Separator\n(You can make a copy of, or modify, this frame)"
            n87 = call <vilib>:"Add State(s) to Queue__jki_lib_state_machine.vi"("State(s) in (\"\")"=w259) -> ("States Out"=w258:string)  [unwired: 14 in]
          }
          frame "Process: Sync" {
            n88 = Unbundle By Name(w267) -> ("Self Reference"=w263:refnum<class "System.lvclass">)
            n89 = call <vilib>:"WaitOnProcessSync.vi"("error in (no error)"=w262, "SMO"=w263) -> ("error out"=w261:errorcluster, "Don't run?"=w266:bool)  [unwired: 7 in, 1 out]
            n90 = Select(t="Data: Cleanup\nEvents: Unregister\nExit", s=w266, f="") -> (s? t:f=w260:string)
            n91 = call <vilib>:"Add State(s) to Queue__jki_lib_state_machine.vi"("State(s) in Front (\"\")"=w260, "State(s) in (\"\")"=w270) -> ("States Out"=w269:string)  [unwired: 13 in]
          }
          frame "---------- Events ----------" {
            # "Template Separator\n(You can make a copy of, or modify, this frame)"
            n92 = call <vilib>:"Add State(s) to Queue__jki_lib_state_machine.vi"("State(s) in (\"\")"=w275) -> ("States Out"=w274:string)  [unwired: 14 in]
          }
          frame "Events: Register" {
            # "Monitor Pump State Events"
            n93 = Unbundle By Name(w288) -> ("Self Reference"=w280:refnum<class "System.lvclass">)
            n94 = call <vilib>:"GetProtectedEvents.vi"("SMO"=w280) -> ("error out"=w283:errorcluster, "SMO Protected Events"=w287:T7)  [unwired: 8 in, 1 out]
            n95 = call "Get System Dependencies.vi"("System in"=w280) -> ("error out"=w276:errorcluster, "Pump"=w279:refnum<class "Pump.lvclass">)  [unwired: 8 in, 1 out]
            n96 = call "Read Pump State Event.vi"("error in (no error)"=w276, "Pump in"=w279) -> ("error out"=w277:errorcluster, "Pump State Event"=w278:refnum<user-event>)  [unwired: 7 in, 1 out]
            n97 = Unbundle By Name(w280) -> ("Pump Setpoint Payload"=w282:refnum<user-event>)
            n98 = register-events(w287, w282, w278) -> (reference out=w281:refnum<event-registration>, error out=w284:errorcluster)  [unwired: 2 in]
            n99 = Merge Errors(w286, w284, w283, w277) -> (w285:errorcluster)
            n100 = call <vilib>:"Add State(s) to Queue__jki_lib_state_machine.vi"("State(s) in (\"\")"=w290) -> ("States Out"=w289:string)  [unwired: 14 in]
          }
          frame "Events: Unregister" {
            n101 = Unregister For Events(event registration refnum=w293, error in=w292) -> (error out=w291:errorcluster)
            n102 = call <vilib>:"Clear Errors.vi"("error in (no error)"=w291) -> ()  [unwired: 5 in, 2 out]
            n103 = call <vilib>:"Add State(s) to Queue__jki_lib_state_machine.vi"("State(s) in (\"\")"=w296) -> ("States Out"=w295:string)  [unwired: 14 in]
          }
          frame "---------- Compute ----------" {
            n104 = call <vilib>:"Add State(s) to Queue__jki_lib_state_machine.vi"("State(s) in (\"\")"=w301) -> ("States Out"=w300:string)  [unwired: 14 in]
          }
        }
      }
    }
    frame Error {
    }
  }
  n105 = call-parent "Process.vi"("error in"=w10, "SMO"=w9) -> ("error out"=w8:errorcluster, "SMO out"=→"System out":refnum<class "System.lvclass">)  [unwired: 8 in]
  n106 = Merge Errors(w8, w7) -> (→"error out":errorcluster)
